vi "update_location.vi"(8 "error in (no error)":errorcluster, 11 "Batch Processing Cluster":T1 {"File Location" items=["Unknown"=-5, "IDL Processing"=-4, "Writing from Queue"=-3, "Labview Files"=-2, "Retry Labview files"=-1, "Local Cache "=0, "Old Storage"=1, "Storage"=2]}) -> (0 "error out":errorcluster, 3 "Test Server":bool)   [LabVIEW 2013]
uses:
  bp_cluster.ctl
  Private/File_location.ctl
  <vilib>/addons/database/NI_Database_API.lvlib
panel:
  out "concatenated string":string
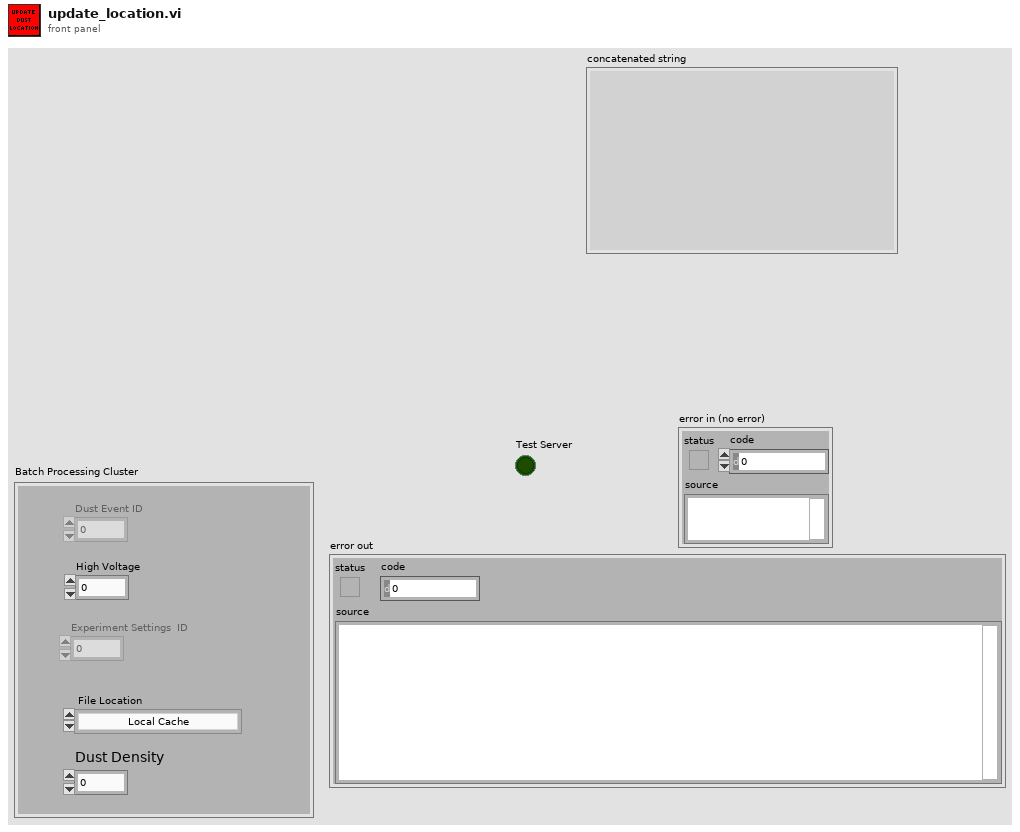
[diagram p1: front panel]
types:
  T1 = typedef "bp_cluster.ctl" = cluster{"Dust Event ID":i64, "High Voltage":sgl, "Experiment Settings  ID":i64, "File Location":T2, "Dust Density":dbl}
  T2 = typedef "File_location.ctl" = i8
  T3 = typedef "NI_Database_API.lvlib/Conn ObjectReference.ctl" = refnum<k1>
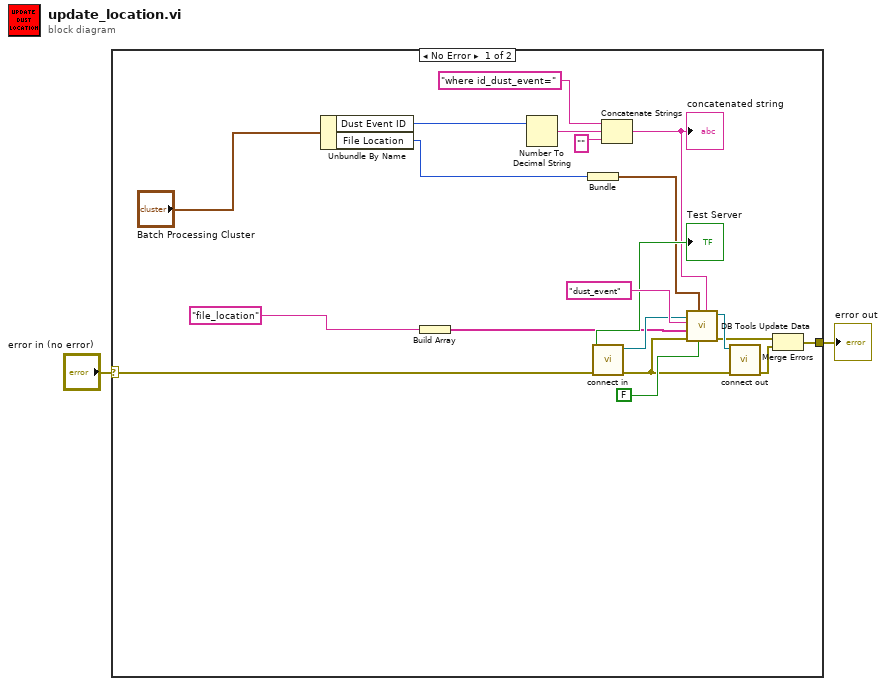
[diagram p0: block diagram]
diagram:
  n1 = case shown="No Error" "error in (no error)" {
    selector: "error in (no error)" -> [w18 w23]
    tunnel: [w15 w23] -> w1
    frame No Error {
      n2 = Unbundle By Name("Batch Processing Cluster") -> ("Dust Event ID"=w11:i64, "File Location"=w3:T2)
      n3 = Build Array("file_location" ("string")) -> (w5:string[])
      n4 = Number To Decimal String(number=w11) -> (decimal integer string=w8:string)  [unwired: 1 in]
      n5 = Bundle("File Location"=w3) -> (w4:cluster{"File Location":T2})  [unwired: 1 in]
      n6 = call "connect in.vi"("error in (no error)"=w18) -> ("error out"=w17:errorcluster, "Database Connection"=w21:T3, "Test Server"=→"Test Server":bool)  [unwired: 6 in]
      n7 = Concatenate Strings("where id_dust_event=" ("condition"), w8, "" ("string")) -> (w10:string)
      "concatenated string" <- w10
      n8 = call <vilib>:"DB Tools Update Data.vi"("condition"=w10, "flatten cluster? (F)"=FALSE ("create table? (F)"), "data"=w4, "error in (no error)"=w17, "columns"=w5, "table"="dust_event", "connection reference"=w21) -> ("error out"=w13:errorcluster, "connection reference out"=w14:T3)  [unwired: 3 in]
      n9 = call "connect out.vi"("error in (no error)"=w17, "connection reference"=w14) -> ("error out"=w16:errorcluster)  [unwired: 9 in]
      n10 = Merge Errors(w13, w16) -> (w15:errorcluster)
    }
    frame Error {
    }
  }
  "error out" <- w1
